vi "Offset Locking- Main v3.0.vi"() -> ()   [LabVIEW 2017]
uses:
  <vilib>/Utility/error.llb/DialogType.ctl
  <vilib>/Analysis/1siggen.llb/Ramp Pattern by Samples.vi
  <vilib>/measure/mamon.llb/Waveform Peak Detection for 1 Chan.vi
  <vilib>/addons/control/pid/pid.llb/PID Advanced (DBL).vi
  <vilib>/measure/NI_MAPro.lvlib
  <vilib>/addons/control/pid/NI_PID_pid.lvlib
  <vilib>/Analysis/NI_AALBase.lvlib
  <vilib>/measure/NI_MABase.lvlib
panel:
  in  "start":dbl format="%0.2f"
  in  "end":dbl=1.0 format="%0.2f"
  in  "samples":i32=128
  in  "Waveform Test?":bool
  in  "reset signal":bool
  in  "phase":dbl format="%.2p"
  out "Chirp Rate":dbl format="%#_g GHz/ms"
  out "Single Mode?":bool
  out "# of Peaks found when Chirping?":i32
  in  "Minimum amplitude for Slave":dbl=0.15 format="%.2p"
  in  "Minimum \namplitude\nfor peaks":dbl=0.5 format="%#_13g V"
  in  "PZT Voltage to \nFrequency Conversion":dbl=-1.41655 format="%#_g V/GHz"
  out "PZT Chirp Output":waveform(dbl)(graph)
  in  "offset":dbl format="%0.2p V"
  in  "Sampling Info":cluster{"Fs":dbl, "#s":dbl}={"Fs"=10000.0, "#s"=100.0} {"Fs" format="%.2p"}
  in  "frequency":dbl=10.0 format="%0.2p Hz"
  in  "Chirp Amplitude":dbl=1.5 format="%0.2p GHz"
  in  "Run Chirp Program?":bool
  out "Run Time (min)":dbl
  out "standard deviation":dbl format="%0.3e"
  in  "Ref Peak 2":i32=1
  in  "Ref Peak":i32=2
  in  "First Cal Peak":i32
  in  "Last Cal Peak":i32=2
  out "# found":i32
  out "Offset":dbl(graph)
  in  "Manual PZT Control":dbl format="%#_g V"
  in  "Engage PZT PID?":bool
  out "Offset (GHz)":dbl format="%#_4g"
  in  "# of Shots for Averaging":i32=100
  in  "Name Convention":string="Chirp Offset Lock Log"
  in  "Save Directory":path=path "C:/Users/LabUser/Google Drive/Measurements"
  out "Four peaks?":bool
  out "PZT Output":dbl(graph)
  in  "PID Gains":T1={"proportional gain (Kc)"=-1.0, "integral time (Ti, min)"=0.01, "derivative time (Td, min)"=0.0} {"derivative time (Td, min)" format="%.3f"; "integral time (Ti, min)" format="%.3f"; "proportional gain (Kc)" format="%.3f"}
  in  "Setpoint Range (GHz)":cluster{"setpoint high":dbl, "setpoint low":dbl}={"setpoint high"=7.7901, "setpoint low"=7.7899} {"setpoint high" format="%.4f"; "setpoint low" format="%.4f"}
  out "dt out (s)":dbl format="%.3f"
  in  "Frequency Offset Setpoint (GHz)":dbl=7.79 format="%.3f"
  out "GHz/sec":dbl
  out "dt":dbl format="%#_4g"
  out "Locations":dbl[](array[numeric]) format="%.2p"
  out "Amplitudes":dbl[](array[numeric]) format="%.2p"
  out "2nd Derivatives":dbl[](array[numeric]) format="%.2p"
  out "10 GHz FPI":dynamicdata(graph)
  in  "Stop":bool
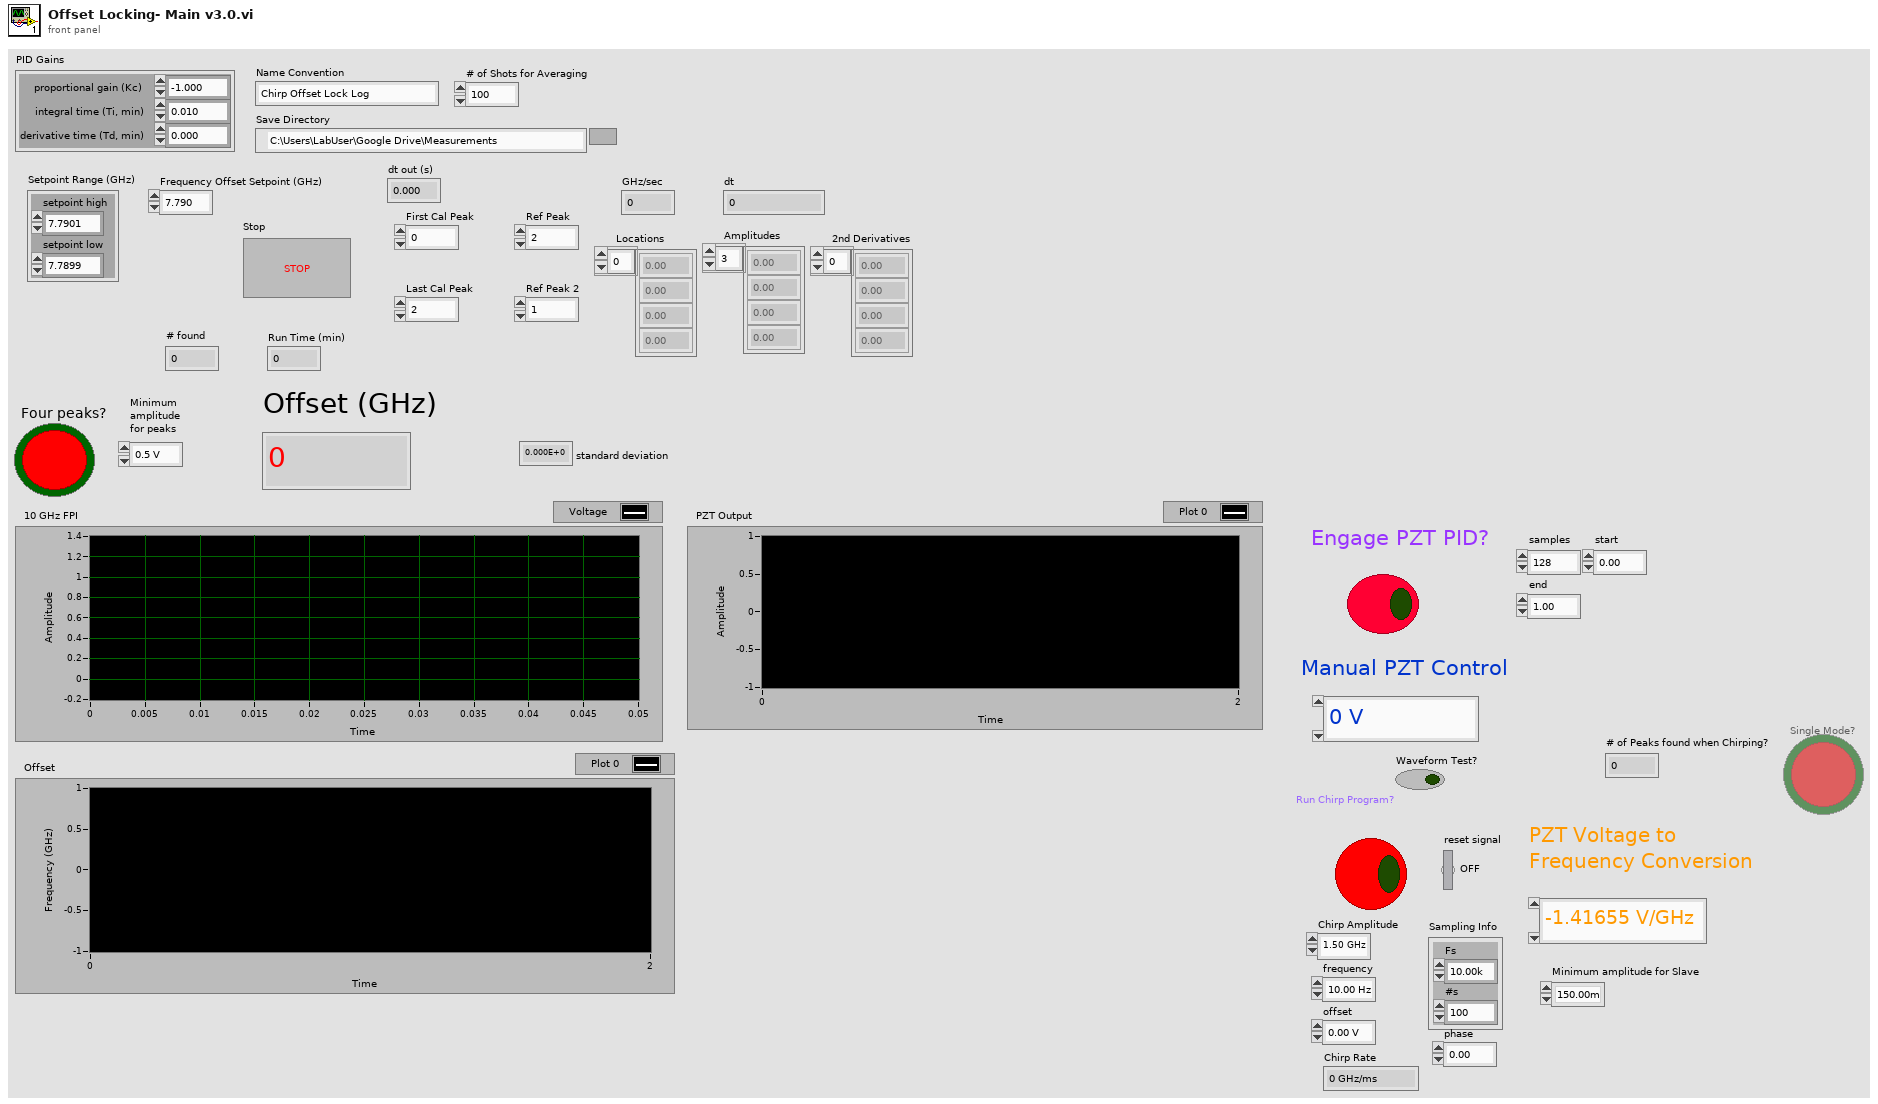
[diagram p1: front panel]
types:
  T1 = cluster{"proportional gain (Kc)":dbl, "integral time (Ti, min)":dbl, "derivative time (Td, min)":dbl}
  T2 = enum8{"Enabled", "Disabled", "Disabled and Grayed Out"}
  T3 = typedef "DialogType.ctl" = u16
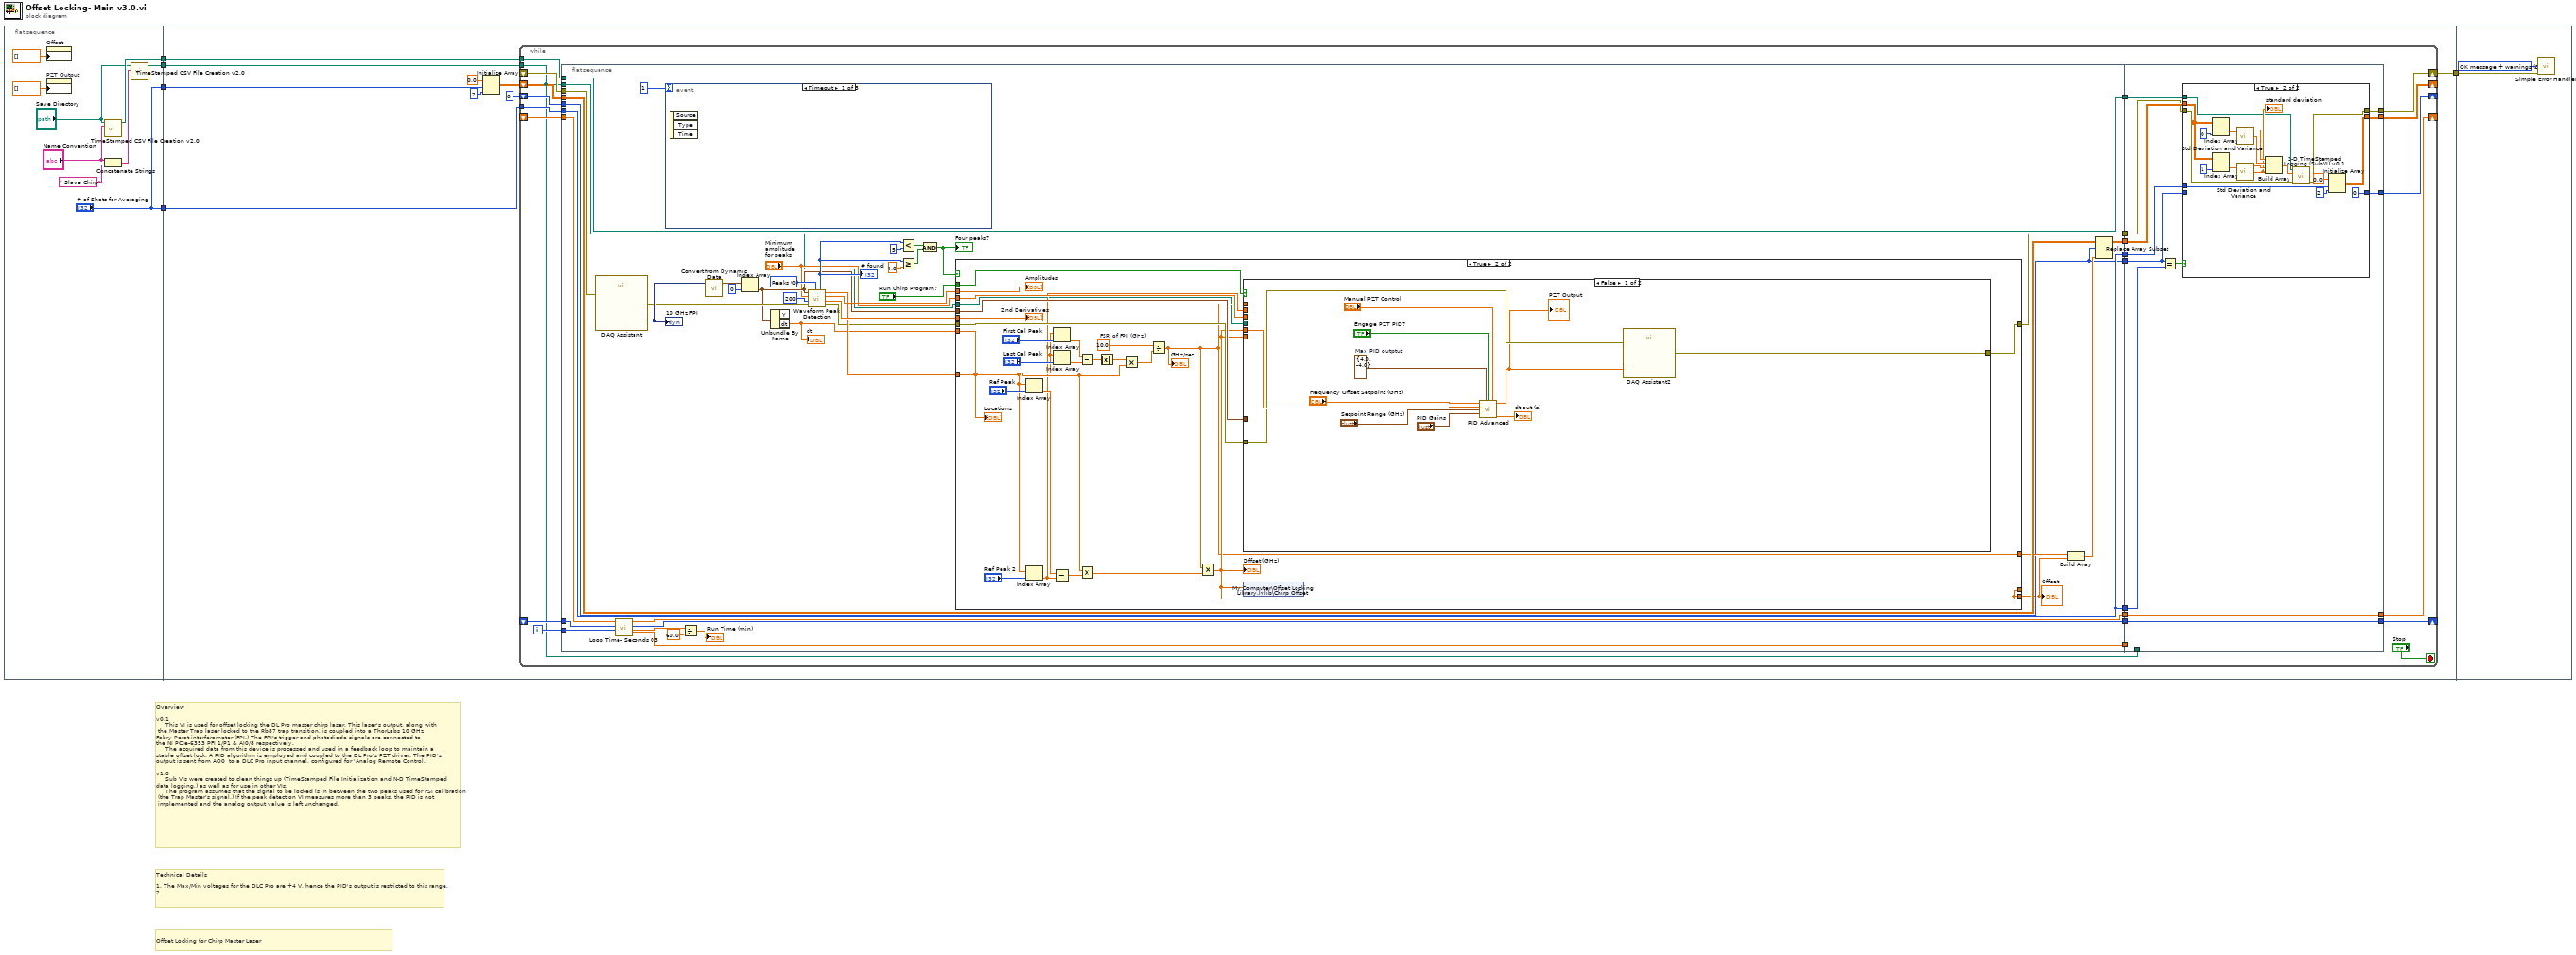
[diagram p0: block diagram]
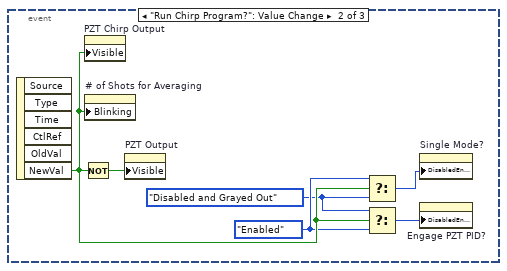
[diagram p2: hidden frame]
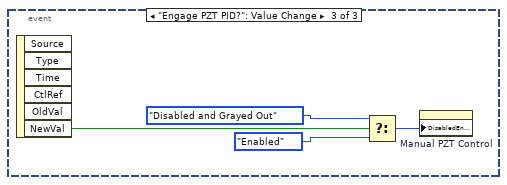
[diagram p3: hidden frame]
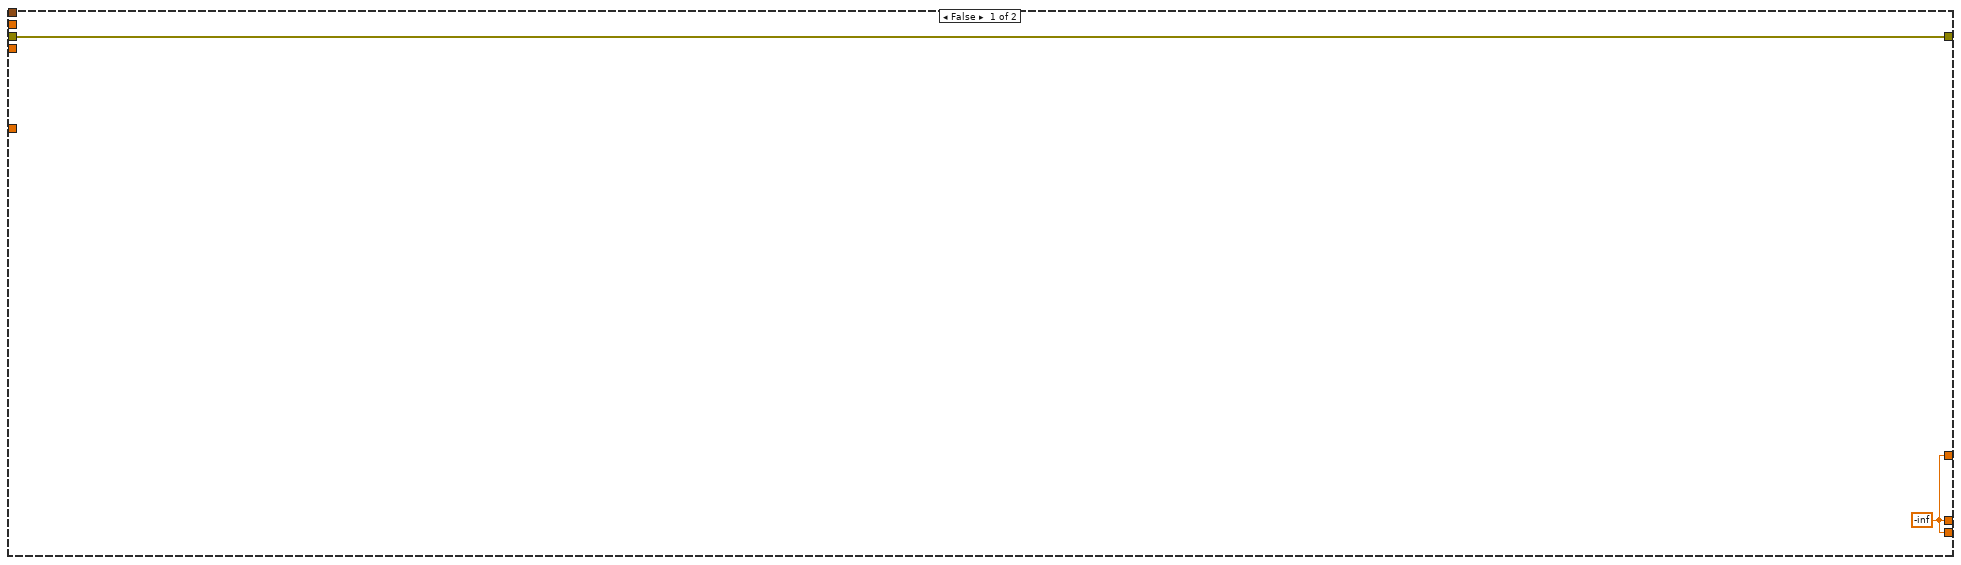
[diagram p4: hidden frame]
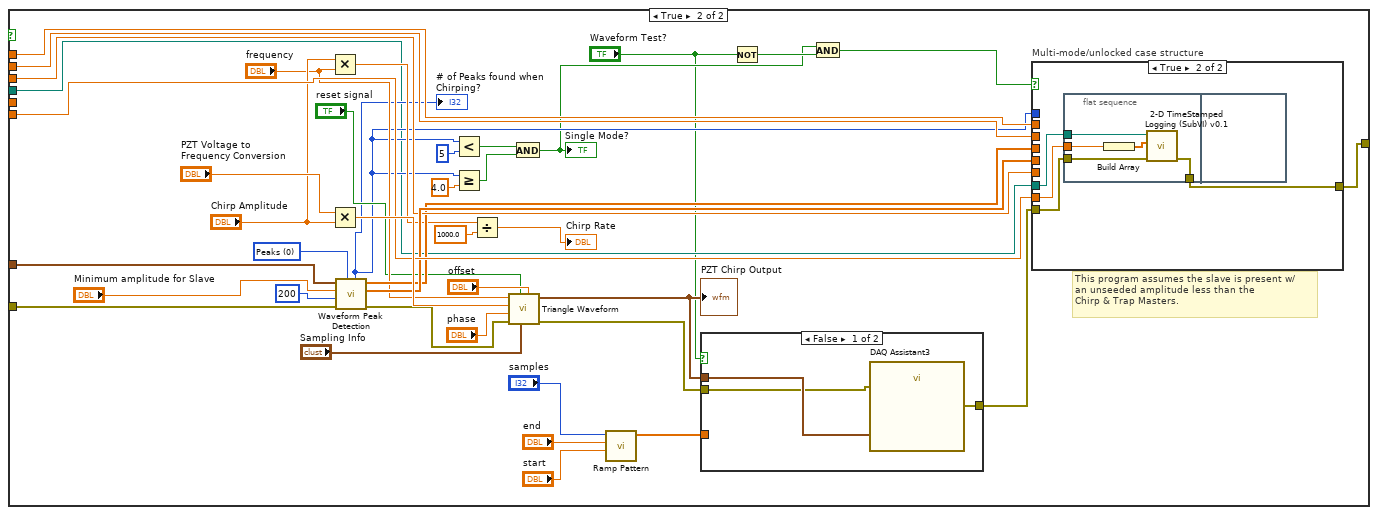
[diagram p5: hidden frame]
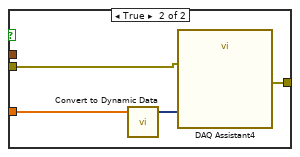
[diagram p6: hidden frame]
diagram:
  # "Technical Details\n\n1. The Max/Min voltages for the DLC Pro are +4 V, hence the PID's output is restricted to this range.\n2."
  # "Overview\n\nv0.1\n     This VI is used for offset locking the DL Pro master chirp laser. This laser's output, along with\n the Master Trap laser locked to the Rb87 trap transition, is coupled into a ThorLabs 10 GHz \nFabry-Perot interferometer (FPI.) The FPI's trigger and photodiode signals are connected to \nthe NI PCIe-6353 PFI 1/P1 & AI0/8 respectively. \n     The acquired data from this device is processed and used in a feedback loop to maintain a \nstable offset lock. A PID algorithm is employed and coupled to the DL Pro's PZT driver. The PID's\noutput is sent from AO0  to a DLC Pro input channel, configured for 'Analog Remote Control.'\n\nv1.0\n     Sub VIs were created to clean things up (TimeStamped File Initialization and N-D TimeStamped \ndata logging,) as well as for use in other VIs.\n     The program assumes that the signal to be locked is in between the two peaks used for FSI calibration\n (the Trap Master's signal.) If the peak detection VI measures more than 3 peaks, the PID is not\n implemented and the analog output value is left unchanged."
  # "Offset Locking for Chirp Master Laser"
  n1 = flat-sequence {
    tunnel: [w14] -> w5
    tunnel: ["# of Shots for Averaging"] -> w3
    tunnel: ["# of Shots for Averaging"] -> w2
    tunnel: [w6] -> w1
    tunnel: w5 -> [w23]
    tunnel: [w22] -> w4
    tunnel: w3 -> [w20]
    tunnel: w2 -> [w17]
    tunnel: w1 -> [w15]
    tunnel: w4 -> [w234]
    frame #0 {
      n2 = property on="Offset" class="WFChart (strict)"("History Data"=dbl[] []) -> ()  [unwired: 2 in, 2 out]
      n3 = property on="PZT Output" class="WFChart (strict)"("History Data"=dbl[] []) -> ()  [unwired: 2 in, 2 out]
      n4 = call "TimeStamped CSV File Creation v2.0.vi"("Name Convention"="Name Convention", "Base Directory"="Save Directory") -> ("path"=w14:path)  [unwired: 8 in, 1 out]
      n5 = Concatenate Strings("Name Convention", " Slave Chirp" ("string")) -> (w8:string)
      n6 = call "TimeStamped CSV File Creation v2.0.vi"("Name Convention"=w8, "Base Directory"="Save Directory") -> ("path"=w6:path)  [unwired: 8 in, 1 out]
    }
    frame #1 {
      n7 = Initialize Array(0.0 ("element"), w17, 2 ("dimension size")) -> (w19:dbl[][])
      n8 = while {
        shift-right: [w35] -> w22
        shift-left: _ -> [w46]
        tunnel: w23 -> [w44]
        shift-right: [w33] -> _
        shift-left: 0 -> [w42]
        tunnel: w20 -> [w40]
        shift-right: [w34] -> _
        shift-left: w19 -> [w37]
        shift-right: [w31] -> _
        shift-left: _ -> [w28]
        shift-right: [w29] -> _
        shift-left: _ -> [w27]
        tunnel: w15 -> [w24]
        i -> [w26]
        stop <- "Stop" stop-if-true
        n9 = flat-sequence {
          tunnel: w46 -> [w77]
          tunnel: [w53] -> w45
          tunnel: w44 -> [w75]
          tunnel: [w75] -> w43
          tunnel: w42 -> [w69]
          tunnel: [w69] -> w41
          tunnel: w40 -> [w70]
          tunnel: [w70] -> w39
          tunnel: [w74] -> w38
          tunnel: w37 -> [w73]
          tunnel: [w70] -> w36
          tunnel: [w68] -> w32
          tunnel: [w67] -> w30
          tunnel: w28 -> [w66]
          tunnel: w27 -> [w65]
          tunnel: w26 -> [w64]
          tunnel: [w56] -> w25
          tunnel: w24 -> [w49]
          tunnel: w45 -> [w207]
          tunnel: w43 -> [w208]
          tunnel: w41 -> [w202]
          tunnel: w39 -> [w212]
          tunnel: w38 -> [w209]
          tunnel: w36 -> [w210]
          tunnel: [w201] -> w35
          tunnel: [w206] -> w34
          tunnel: [w205] -> w33
          tunnel: w32 -> [w204]
          tunnel: [w204] -> w31
          tunnel: [w203] -> w29
          tunnel: w30 -> [w203]
          tunnel: w25 -> [_]
          tunnel: w24 -> [_]
          frame #0 {
            w79 = u16 0 items=["Peaks", "Valleys"] ("peaks/valleys")
            n10 = call "DAQ Assistant"("error in"=w77) -> ("data"=w85:dynamicdata, "error out"=w76:errorcluster)  [unwired: 16 in, 1 out]
            "10 GHz FPI" <- w85
            n11 = call "Loop Time- Seconds 03.vi"("Loop Iteration"=w64, "Shift Registered Time In"=w65, "Shift Registered In"=w66) -> ("t"=w56:dbl, "Shift Registered Time Out"=w67:u32, "Shift Registered Out"=w68:dbl)  [unwired: 6 in]
            n12 = event shown="[0] Timeout" {
              selector: _ -> [_ _ _]
              dyn-events: _ -> [_ _ _]
              timeout: 1 -> [_ _ _]
              event Timeout {
                n13 = event-data() -> ()  [unwired: 1 in, 3 out]
              }
              event "Run Chirp Program?": Value Change {
                w89 = T2."Enabled" ("Disabled")
                w88 = T2."Disabled and Grayed Out" ("Disabled")
                n14 = event-data() -> ("NewVal"=w91:bool)  [unwired: 1 in, 5 out]
                n15 = Not(x=w91) -> (.not. x?=w92:bool)
                n16 = property on="PZT Chirp Output" class="WFGraph (strict)"("Visible"=w91) -> ()  [unwired: 2 in, 2 out]
                n17 = property on="# of Shots for Averaging" class="DigNum (strict)"("Blinking"=w91) -> ()  [unwired: 2 in, 2 out]
                n18 = property on="PZT Output" class="WFChart (strict)"("Visible"=w92) -> ()  [unwired: 2 in, 2 out]
                n19 = Select(t=w89, s=w91, f=w88) -> (s? t:f=w90:T2)
                n20 = Select(t=w88, s=w91, f=w89) -> (s? t:f=w93:T2)
                n21 = property on="Single Mode?" class="Bool (strict)"("DisabledEnum"=w90) -> ()  [unwired: 2 in, 2 out]
                n22 = property on="Engage PZT PID?" class="Bool (strict)"("DisabledEnum"=w93) -> ()  [unwired: 2 in, 2 out]
              }
              event "Engage PZT PID?": Value Change {
                n23 = event-data() -> ("NewVal"=w97:bool)  [unwired: 1 in, 5 out]
                n24 = Select(t=T2."Disabled and Grayed Out" ("Disabled"), s=w97, f=T2."Enabled" ("Disabled")) -> (s? t:f=w95:T2)
                n25 = property on="Manual PZT Control" class="DigNum (strict)"("DisabledEnum"=w95) -> ()  [unwired: 2 in, 2 out]
              }
            }
            n26 = Divide(x=w56, y=60.0) -> (x/y=→"Run Time (min)":dbl)
            n27 = call "Convert from Dynamic Data"("Dynamic Data Type"=w85) -> ("Array of Waveform"=w87:waveform(dbl)[])  [unwired: 3 in]
            n28 = Index Array(array=w87, index=0) -> (element=w51:waveform(dbl))
            n29 = Unbundle By Name(w51) -> ("dt"=w81:dbl)  [unwired: 1 out]
            "dt" <- w81
            n30 = call-poly <vilib>:"Waveform Peak Detection.vi"("peaks/valleys"=w79, "error in"=w76, "width"=200, "threshold"="Minimum \namplitude\nfor peaks", "Signal In"=w51) -> ("error out"=w54:errorcluster, "2nd Derivatives"=w83:dbl[], "Amplitudes"=w84:dbl[], "Locations"=w82:dbl[], "# found"=w61:i32)  [unwired: 2 in]
            "# found" <- w61
            n31 = Less?(x=w61, y=5) -> (x < y?=w59:bool)
            n32 = Greater Or Equal?(x=w61, y=4.0) -> (x >= y?=w62:bool)
            n33 = And(x=w59, y=w62) -> (x .and. y?=w58:bool)
            "Four peaks?" <- w58
            n34 = case shown="True" w58 {
              tunnel: w84 -> [_ w104]
              tunnel: w83 -> [_ w125]
              tunnel: w82 -> [_ w110]
              tunnel: w81 -> [_ w116]
              tunnel: [w99 w101] -> w72
              tunnel: [w99 w105] -> w63
              tunnel: [w99 w105] -> _
              tunnel: w54 -> [w98 w109]
              tunnel: [w98 w108] -> w53
              tunnel: "Run Chirp Program?" -> [_ w107]
              tunnel: w51 -> [_ w106]
              tunnel: "Minimum \namplitude\nfor peaks" -> [_ w103]
              tunnel: w49 -> [_ w100]
              frame False {
                w99 = -inf
              }
              frame True {
                w123 = 10.0  # FSR of FPI (GHz)
                n35 = Index Array(array=w110, index="Ref Peak") -> (element=w118:dbl)
                n36 = Index Array(array=w110, index="Ref Peak 2") -> (element=w102:dbl)
                n37 = Subtract(x=w118, y=w102) -> (x-y=w117:dbl)
                n38 = Index Array(array=w110, index="First Cal Peak") -> (element=w119:dbl)
                n39 = Index Array(array=w110, index="Last Cal Peak") -> (element=w124:dbl)
                n40 = Subtract(x=w119, y=w124) -> (x-y=w121:dbl)
                n41 = Multiply(x=w116, y=w117) -> (x*y=w115:dbl)
                n42 = Absolute Value(x=w121) -> (abs(x)=w120:dbl)
                n43 = Multiply(x=w120, y=w116) -> (x*y=w122:dbl)
                n44 = Divide(x=w123, y=w122) -> (x/y=w101:dbl)
                "GHz/sec" <- w101
                n45 = Multiply(x=w101, y=w115) -> (x*y=w105:dbl)
                "Offset (GHz)" <- w105
                n46 = case shown="False" w107 {
                  tunnel: w105 -> [w129 _]
                  tunnel: w109 -> [w128 w171]
                  tunnel: [w127 w145] -> w108
                  tunnel: w106 -> [_ w172]
                  tunnel: w105 -> [_ w168]
                  tunnel: w103 -> [_ w162]
                  tunnel: w102 -> [_ w160]
                  tunnel: w101 -> [_ w159]
                  tunnel: w100 -> [_ w147]
                  frame False {
                    w132 = cluster{"output high":dbl, "output low":dbl} {"output high"=4.0, "output low"=-4.0}  # Max PID outptut
                    n47 = call-poly <vilib>:"PID Advanced.vi"("setpoint"="Frequency Offset Setpoint (GHz)", "output range"=w132, "auto? (T)"="Engage PZT PID?", "manual control"="Manual PZT Control", "process variable"=w129, "setpoint range"="Setpoint Range (GHz)", "PID gains"="PID Gains") -> ("output"=w126:dbl, "dt out (s)"=→"dt out (s)":dbl)  [unwired: 7 in]
                    "PZT Output" <- w126
                    n48 = call "DAQ Assistant2"("data"=w126, "error in"=w128) -> ("error out"=w127:errorcluster)  [unwired: 16 in, 1 out]
                  }
                  frame True {
                    w158 = u16 0 items=["Peaks", "Valleys"] ("peaks/valleys")
                    # "This program assumes the slave is present w/ \nan unseeded amplitude less than the \nChirp & Trap Masters."
                    n49 = Multiply(x="Chirp Amplitude", y="frequency") -> (x*y=w154:dbl)
                    n50 = Multiply(x="PZT Voltage to \nFrequency Conversion", y="Chirp Amplitude") -> (x*y=w174:dbl)
                    n51 = call-poly <vilib>:"Waveform Peak Detection.vi"("peaks/valleys"=w158, "error in"=w171, "width"=200, "threshold"="Minimum amplitude for Slave", "Signal In"=w172) -> ("error out"=w170:errorcluster, "Amplitudes"=w163:dbl[], "Locations"=w161:dbl[], "# found"=w148:i32)  [unwired: 2 in, 1 out]
                    "# of Peaks found when Chirping?" <- w148
                    n52 = Less?(x=w148, y=5) -> (x < y?=w164:bool)
                    n53 = Greater Or Equal?(x=w148, y=4.0) -> (x >= y?=w166:bool)
                    n54 = Divide(x=w154, y=1000.0) -> (x/y=→"Chirp Rate":dbl)
                    n55 = call <vilib>:"Triangle Waveform.vi"("offset"="offset", "sampling info"="Sampling Info", "reset signal"="reset signal", "error in (no error)"=w170, "phase"="phase", "amplitude"=w174, "frequency"="frequency") -> ("error out"=w149:errorcluster, "signal out"=w150:waveform(dbl))  [unwired: 3 in]
                    "PZT Chirp Output" <- w150
                    n56 = And(x=w164, y=w166) -> (x .and. y?=w143:bool)
                    "Single Mode?" <- w143
                    n57 = call-poly <vilib>:"Ramp Pattern.vi"("start"="start", "end"="end", "samples"="samples") -> ("Ramp Pattern"=w140:dbl[])  [unwired: 7 in, 1 out]
                    n58 = case shown="False" "Waveform Test?" {
                      tunnel: w150 -> [w180 _]
                      tunnel: w149 -> [w179 w184]
                      tunnel: [w178 w183] -> w146
                      tunnel: w140 -> [_ w182]
                      frame False {
                        n59 = call "DAQ Assistant3"("data"=w180, "error in"=w179) -> ("error out"=w178:errorcluster)  [unwired: 16 in, 1 out]
                      }
                      frame True {
                        n60 = call "Convert to Dynamic Data"("Array"=w182) -> ("Dynamic Data Type"=w181:dynamicdata)  [unwired: 3 in]
                        n61 = call "DAQ Assistant4"("data"=w181, "error in"=w184) -> ("error out"=w183:errorcluster)  [unwired: 16 in, 1 out]
                      }
                    }
                    n62 = Not(x="Waveform Test?") -> (.not. x?=w144:bool)
                    n63 = And(x=w143, y=w144) -> (x .and. y?=w142:bool)
                    n64 = case "Multi-mode/unlocked case structure" shown="True" w142 {
                      tunnel: w168 -> [_ w195]
                      tunnel: w148 -> [w191 _]
                      tunnel: w163 -> [w190 _]
                      tunnel: w162 -> [w189 _]
                      tunnel: w161 -> [w188 _]
                      tunnel: w160 -> [w187 _]
                      tunnel: w159 -> [w186 _]
                      tunnel: w147 -> [_ w194]
                      tunnel: w146 -> [w185 w193]
                      tunnel: [w185 w192] -> w145
                      frame False {
                        n65 = for {
                          N: w191 -> [_]
                          tunnel: w190 -> [_] mode=indexing
                          tunnel: w189 -> [_]
                          tunnel: w188 -> [_] mode=indexing
                          tunnel: w187 -> [_]
                          tunnel: w186 -> [_]
                        }
                      }
                      frame True {
                        n66 = flat-sequence {
                          tunnel: w195 -> [w200]
                          tunnel: w194 -> [w198]
                          tunnel: w193 -> [w197]
                          tunnel: [w196] -> w192
                          frame #0 {
                            n67 = Build Array(w200) -> (w199:dbl[])
                            n68 = call "2-D TimeStamped Logging (SubVI) v0.1.vi"("error in (no error)"=w197, "array"=w199, "path"=w198) -> ("error out"=w196:errorcluster)  [unwired: 8 in]
                          }
                          frame #1 {
                          }
                        }
                      }
                    }
                  }
                }
                n69 = shared-variable "My Computer\\Offset Locking Library.lvlib\\Chirp Offset"(w105) -> ()  [unwired: 1 in, 1 out]
                "2nd Derivatives" <- w125
                "Amplitudes" <- w104
                "Locations" <- w110
              }
            }
            "Offset" <- w63
            n70 = Build Array(w72, w63) -> (w71:dbl[])
            n71 = Replace Array Subset(array=w73, new element=w71, index (row)=w69) -> (w74:dbl[][])  [unwired: 1 in]
          }
          frame #1 {
            n72 = Equal?(x=w202, y=w212) -> (x = y?=w211:bool)
            n73 = case shown="True" w211 {
              tunnel: w210 -> [_ w216]
              tunnel: w209 -> [w215 w229]
              tunnel: w208 -> [_ w223]
              tunnel: w207 -> [w213 w222]
              tunnel: [w215 w219] -> w206
              tunnel: w202 -> [w214 _]
              tunnel: [w214 0] -> w205
              tunnel: [w213 w217] -> w201
              frame False {
              }
              frame True {
                n74 = Index Array(array=w229, index (col)=0 ("disabled index (col)")) -> (element=w232:dbl[])  [unwired: 1 in]
                n75 = Index Array(array=w229, index (col)=1 ("disabled index (col)")) -> (element=w230:dbl[])  [unwired: 1 in]
                n76 = call <vilib>:"Std Deviation and Variance.vi"("X"=w232) -> ("mean"=w228:dbl, "standard deviation"=w227:dbl)  [unwired: 1 in, 1 out]
                n77 = call <vilib>:"Std Deviation and Variance.vi"("X"=w230) -> ("mean"=w226:dbl, "standard deviation"=w225:dbl)  [unwired: 1 in, 1 out]
                "standard deviation" <- w225
                n78 = Build Array(w228, w227, w226, w225) -> (w224:dbl[])
                n79 = call "2-D TimeStamped Logging (SubVI) v0.1.vi"("error in (no error)"=w222, "array"=w224, "path"=w223) -> ("error out"=w217:errorcluster)  [unwired: 8 in]
                n80 = Initialize Array(0.0 ("element"), w216, 2 ("dimension size")) -> (w219:dbl[][])
              }
            }
          }
        }
      }
    }
    frame #2 {
      w235 = T3 3 items=["no dialog", "OK message", "continue or stop message", "OK message + warnings", "continue/stop + warnings"] ("type of dialog (OK msg:1)")
      n81 = call <vilib>:"Simple Error Handler.vi"("type of dialog (OK msg:1)"=w235, "error in (no error)"=w234) -> ()  [unwired: 3 in, 5 out]
    }
  }
